vi "LVClass_HasoSlopes ctor from HasoConfig.vi"(0 "HasoSlopes (const)":refnum<class "HasoSlopes.lvclass">, 5 "HasoConfig":refnum<class "HasoConfig.lvclass">, 11 "error in (no error)":errorcluster) -> (4 "HasoSlopes (new)":refnum<class "HasoSlopes.lvclass">, 15 "error out":errorcluster)   [LabVIEW 2020, in "HasoSlopes.lvclass"]
uses:
  HasoSlopes.lvclass
  HasoConfig.lvclass
  Handle creation.ctl
  HasoSlopes.lvclass/HasoSlopes.ctl
  LVClasse_HasoConfig Read HasoConfig.vi
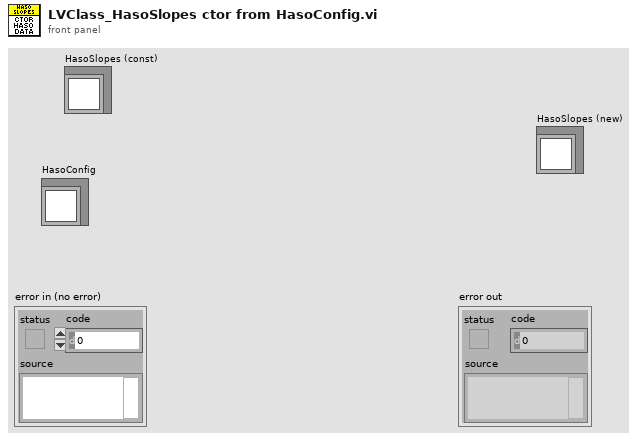
[diagram p1: front panel]
types:
  T1 = typedef "Handle creation.ctl" = enum16{"By ctor", "By write function"}
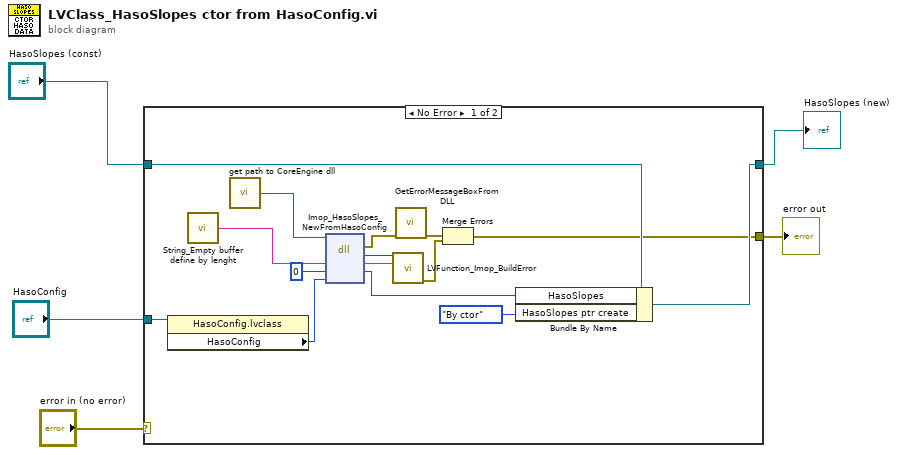
[diagram p0: block diagram]
diagram:
  n1 = case shown="No Error" "error in (no error)" {
    selector: "error in (no error)" -> [_ w22]
    tunnel: [w6 w22] -> w4
    tunnel: [w14 w21] -> w1
    tunnel: "HasoSlopes (const)" -> [w15 w21]
    tunnel: "HasoConfig" -> [w10 _]
    frame No Error {
      n2 = property class="HasoConfig.lvclass"(reference=w10) -> ("HasoConfig"=w9:i32)  [unwired: 1 in, 2 out]
      n3 = call "String_Empty buffer define by lenght.vi"() -> ("Empty buffer"=w16:string)  [unwired: 1 in]
      n4 = call "get path to CoreEngine dll.vi"() -> ("path to wavekit library"=w13:path)  [unwired: 14 in, 1 out]
      n5 = dll-call lib="D:/FLE/0.Code/CoreEngine4_Suite/LV2011_interface/DLLs/c_interface_vc100.dll" fn="Imop_HasoSlopes_NewFromHasoConfig"(path in=w13, "message"=w16, "objet"=0, "HasoConfig"=w9) -> (error out=w12:errorcluster, "return type"=w19:i32, "message"=w18:string, "objet"=w17:i64)  [unwired: 3 in, 1 out]
      n6 = call "LVFunction_Imop_BuildError.vi"("code"=w19, "String to Prepend to source (\"\")"=w18) -> ("error out"=w7:errorcluster)  [unwired: 13 in]
      n7 = call "GetErrorMessageBoxFromDLL.vi"("error IN"=w12) -> ("error OUT"=w8:errorcluster)  [unwired: 10 in]
      n8 = Merge Errors(w8, w7) -> (w6:errorcluster)
      n9 = Bundle By Name(cluster=w15, "HasoSlopes"=w17, "HasoSlopes ptr create"=Handle_creation."By ctor" ("HasoData ptr create")) -> (w14:refnum<class "HasoSlopes.lvclass">)
    }
    frame Error {
    }
  }
  "error out" <- w4
  "HasoSlopes (new)" <- w1
